vi "Syringe Heater Interlock Configuration.vi"(8 "error in (no error)":errorcluster, 11 "cRIO-CO2 in":refnum<class "cRIO-CO2.lvclass">) -> (0 "error out":errorcluster, 2 "Interlock Chain":refnum<class "Interlock Chain.lvclass">, 3 "cRIO-CO2 out":refnum<class "cRIO-CO2.lvclass">)   [LabVIEW 2015, in "cRIO-Carbondioxide.lvlib" / "cRIO-CO2.lvlib" / "cRIO-CO2.lvclass"]
uses:
  cRIO-CO2.lvclass
  Interlocks/Interlock Chain/Interlock Chain.lvclass
  Interlocks/Interlock/Interlock.lvclass
  Interlocks/Interlock DBL/Range/Interlock Range.lvclass
  Interlocks/Interlock Bool/Interlock Bool.lvclass
  cRIO-CO2.lvclass/cRIO-CO2.ctl
  Interlocks/Interlock Bool/Interlock Bool.lvclass/Interlock Bool.ctl
  Interlocks/Interlock DBL/Range/Interlock Range.lvclass/Interlock Range.ctl
  Interlocks/Interlock/Interlock.lvclass/Interlock.ctl
  Interlocks/Interlock Chain/Interlock Chain.lvclass/Interlock Chain.ctl
  Interlocks/IL Action/IL Action.lvclass
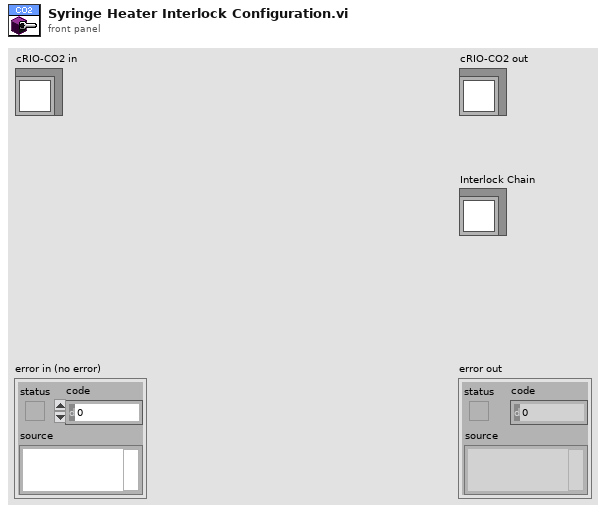
[diagram p1: front panel]
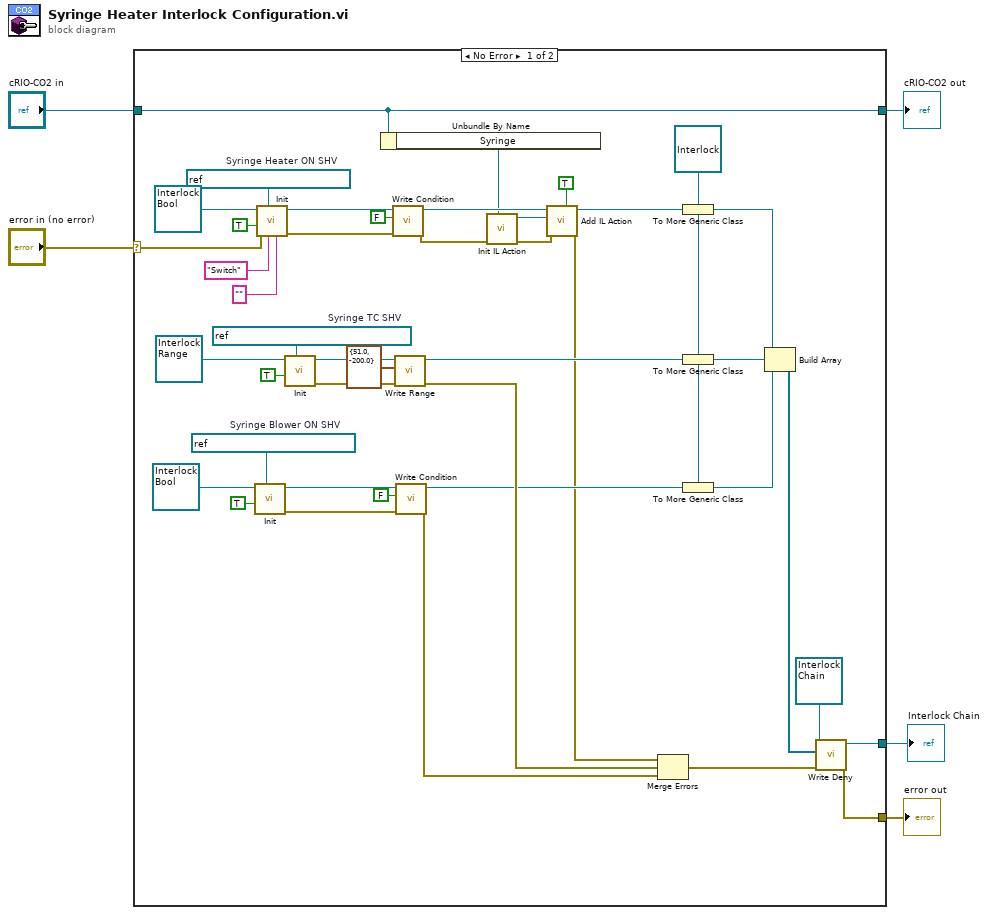
[diagram p0: block diagram]
diagram:
  n1 = case shown="No Error" "error in (no error)" {
    selector: "error in (no error)" -> [w39 w50]
    tunnel: [w35 w50] -> w4
    tunnel: [w17 w49] -> w2
    tunnel: "cRIO-CO2 in" -> [w17 w49]
    tunnel: [w33 _] -> w1
    frame No Error {
      w31 = refnum<k21> "ni.var.psp://crio-carbondioxide/AMS Gas SHV/Blowers/Syringe Blower"  # Syringe Blower ON SHV
      w41 = refnum<k21> "ni.var.psp://10.2.0.20/AMS Gas SHV/Heaters/Syringe Heater ON"  # Syringe Heater ON SHV
      w46 = refnum<k21> "ni.var.psp://crio-carbondioxide/AMS Gas SHV/Gauges/Syringe TC"  # Syringe TC SHV
      w21 = refnum<class "Interlock.lvclass"> refnum ("Interlock.lvclass")
      n2 = call-dynamic "Init.vi"("SHV"=w31, "Stop Self on IL? (T)"=TRUE, "Interlock in"=refnum<class "Interlock Bool.lvclass"> refnum ("Interlock Bool.lvclass")) -> ("error out"=w29:errorcluster, "Interlock out"=w30:refnum<class "Interlock Bool.lvclass">)  [unwired: 7 in]
      n3 = call-dynamic "Init.vi"("Interlock message (\" -> Interlock!\")"="" ("Interlock message (\" -> Interlock!\")"), "Name (SHV Name if empty)"="Switch", "SHV"=w41, "error in (no error)"=w39, "Stop Self on IL? (T)"=TRUE, "Interlock in"=refnum<class "Interlock Bool.lvclass"> refnum ("Interlock Bool.lvclass")) -> ("error out"=w27:errorcluster, "Interlock out"=w42:refnum<class "Interlock Bool.lvclass">)  [unwired: 4 in]
      n4 = call-dynamic "Init.vi"("SHV"=w46, "Stop Self on IL? (T)"=TRUE, "Interlock in"=refnum<class "Interlock Range.lvclass"> refnum ("Interlock DBL.lvclass")) -> ("error out"=w26:errorcluster, "Interlock out"=w47:refnum<class "Interlock Range.lvclass">)  [unwired: 7 in]
      n5 = Unbundle By Name(w17) -> ("Syringe"=w9:refnum<class "Message Enqueuer.lvclass">)
      n6 = call "Write Condition.vi"("error in (no error)"=w27, "Interlock Condition"=FALSE, "Interlock Bool in"=w42) -> ("error out"=w10:errorcluster, "Interlock Bool out"=w16:refnum<class "Interlock Bool.lvclass">)  [unwired: 7 in]
      n7 = call "Write Range.vi"("error in (no error)"=w26, "Range"=cluster{"Upper Limit":dbl, "Lower Limit":dbl} {"Upper Limit"=51.0, "Lower Limit"=-200.0}, "Interlock Bool in"=w47) -> ("error out"=w25:errorcluster, "Interlock Bool out"=w44:refnum<class "Interlock Range.lvclass">)  [unwired: 7 in]
      n8 = call "Write Condition.vi"("error in (no error)"=w29, "Interlock Condition"=FALSE, "Interlock Bool in"=w30) -> ("error out"=w24:errorcluster, "Interlock Bool out"=w22:refnum<class "Interlock Bool.lvclass">)  [unwired: 7 in]
      n9 = call "Init IL Action.vi"("Destination Enqueuer (Default)"=w9, "error in (no error)"=w10) -> ("error out"=w12:errorcluster, "IL Action out"=w11:refnum<class "IL Action.lvclass">)  [unwired: 8 in]
      n10 = call "Add IL Action.vi"("Insert infront (F)"=TRUE, "error in (no error)"=w12, "IL Action in"=w11, "Interlock in"=w16) -> ("error out"=w15:errorcluster, "Interlock out"=w14:refnum<class "Interlock Bool.lvclass">)  [unwired: 6 in]
      n11 = Merge Errors(w15, w25, w24) -> (w23:errorcluster)
      n12 = To More Generic Class(target class=w21, reference=w14) -> (generic class reference=w37:refnum<class "Interlock.lvclass">)
      n13 = To More Generic Class(target class=w21, reference=w44) -> (generic class reference=w20:refnum<class "Interlock.lvclass">)
      n14 = To More Generic Class(target class=w21, reference=w22) -> (generic class reference=w19:refnum<class "Interlock.lvclass">)
      n15 = Build Array(w37, w20, w19) -> (w34:refnum<class "Interlock.lvclass">[])
      n16 = call "Write Deny.vi"("error in (no error)"=w23, "Deny"=w34, "Interlock Chain in"=refnum<class "Interlock Chain.lvclass"> refnum) -> ("error out"=w35:errorcluster, "Interlock Chain out"=w33:refnum<class "Interlock Chain.lvclass">)  [unwired: 7 in]
    }
    frame Error {
    }
  }
  "error out" <- w4
  "cRIO-CO2 out" <- w2
  "Interlock Chain" <- w1
